vi "global.vi"() -> ()   [LabVIEW 2017]
panel:
  in  "Angle":dbl
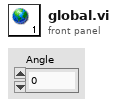
[diagram p1: front panel]
diagram:
